vi "Peak_RAZOFF.vi"(8 "errin":errorcluster) -> (0 "sortie d'erreur":errorcluster caption="errout")   [LabVIEW 2020]
uses:
  PCAN Basic/Controls/BaudrateEenum.ctl
  PCAN Basic/Controls/Channel.ctl
  PCAN Basic/PCANBasic.lvlib
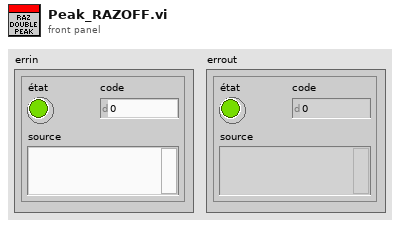
[diagram p1: front panel]
types:
  T1 = typedef "PCANBasic.lvlib/Channel.ctl" = enum16{"PCAN_NONEBUS", "not used1", "not used2", "not used3", "not used4", "not used5", "not used6", "not used7", "not used8", "not used9", "not used10", "not used11", "not used12", "not used13", "not used14", "not used15", "not used16", "not used17", "not used18", "not used19", "not used20", "not used21", "not used22", "not used23", "not used24", "not used25", "not used26", "not used27", "not used28", "not used29", "not used30", "not used31", "not used32", "PCAN_ISABUS1", "PCAN_ISABUS2", "PCAN_ISABUS3", "PCAN_ISABUS4", "PCAN_ISABUS5", "PCAN_ISABUS6", "PCAN_ISABUS7", "PCAN_ISABUS8", "not used41", "not used42", "not used43", "not used44", "not used45", "not used46", "not used47", "not used48", "PCAN_DNGBUS1", "not used50", "not used51", "not used52", "not used53", "not used54", "not used55", "not used56", "not used57", "not used58", "not used59", "not used60", "not used61", "not used62", "not used63", "not used64", "PCAN_PCIBUS1", "PCAN_PCIBUS2", "PCAN_PCIBUS3", "PCAN_PCIBUS4", "PCAN_PCIBUS5", "PCAN_PCIBUS6", "PCAN_PCIBUS7", "PCAN_PCIBUS8", "not used73", "not used74", "not used75", "not used76", "not used77", "not used78", "not used79", "not used80", "PCAN_USBBUS1", "PCAN_USBBUS2", "PCAN_USBBUS3", "PCAN_USBBUS4", "PCAN_USBBUS5", "PCAN_USBBUS6", "PCAN_USBBUS7", "PCAN_USBBUS8", "Not used89", "Not used90", "Not used91", "Not used92", "Not used93", "Not used94", "Not used95", "Not used96", "PCAN_PCCBUS1", "PCAN_PCCBUS2"}
  T2 = typedef "PCANBasic.lvlib/BaudrateEenum.ctl" = enum16{"CAN_Baud_1M", "CAN_Baud_800K", "CAN_BAUD_500K", "CAN_BAUD_250K", "CAN_BAUD_125K", "CAN_BAUD_100K", "CAN_BAUD_95K", "CAN_BAUD_83K", "CAN_BAUD_50K", "CAN_BAUD_47K", "CAN_BAUD_33K", "CAN_BAUD_20K", "CAN_BAUD_10K", "CAN_BAUD_5K", "User Baudrate"}
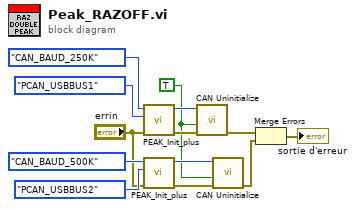
[diagram p0: block diagram]
diagram:
  w2 = TRUE ("Ignore input error")
  n1 = call "PEAK_Init_plus.vi"("errin"="errin", "Channel"=Channel."PCAN_USBBUS1", "BTR0BTR1"=BaudrateEenum."CAN_BAUD_250K") -> ("errout"=w11:errorcluster, "Channel out"=w10:T1)  [unwired: 7 in]
  n2 = call "PEAK_Init_plus.vi"("errin"="errin", "Channel"=Channel."PCAN_USBBUS2", "BTR0BTR1"=BaudrateEenum."CAN_BAUD_500K") -> ("errout"=w1:errorcluster, "Channel out"=w3:T1)  [unwired: 7 in]
  n3 = call "CAN Uninitialize.vi"("error in (no error)"=w11, "Ignore input error"=w2, "Channel"=w10) -> ("error out"=w6:errorcluster)  [unwired: 6 in, 2 out]
  n4 = call "CAN Uninitialize.vi"("error in (no error)"=w1, "Ignore input error"=w2, "Channel"=w3) -> ("error out"=w5:errorcluster)  [unwired: 6 in, 2 out]
  n5 = Merge Errors(w6, w5) -> (→"sortie d'erreur":errorcluster)
